vi "PostCopyScripting.vi"(10 "MetaDataObj":refnum<class "MetaDataObj.lvclass">, 11 "User Project":refnum<vi>) -> ()   [LabVIEW 2020, in "ADAS_IO_Template_MDO.lvclass"]
uses:
  ADAS_IO_Template_MDO.lvclass
  <resource>/dialog/NewProjectWizard/MetaDataObj/MetaDataObj.lvclass
  C:/Program Files/National Instruments/LabVIEW 2020/resource/dialog/NewProjectWizard/MetaDataObj/MetaDataObj.lvclass
  <resource>/dialog/NewProjectWizard/MetaDataObj/MetaDataObj.lvclass/MetaDataObj.ctl
  <resource>/dialog/NewProjectWizard/MetaDataObj/Accessors/Read Project Name.vi
  <resource>/dialog/NewProjectWizard/MetaDataObj/Accessors/Read Project Root.vi
  <resource>/dialog/NewProjectWizard/MetaDataObj/Accessors/Read Overlay Pixmap.vi
  <vilib>/LabVIEW Icon API/lv_icon/Classes/Icon/Icon.lvclass
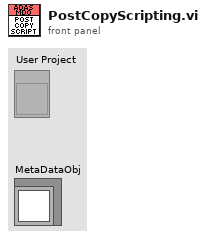
[diagram p1: front panel]
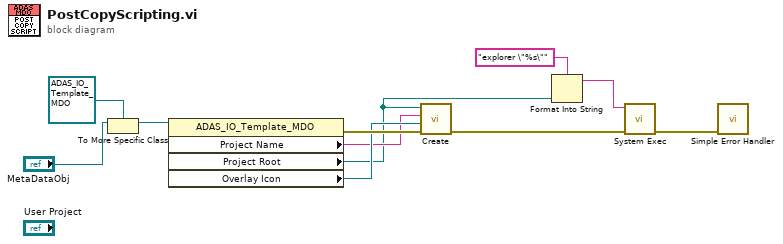
[diagram p0: block diagram]
diagram:
  n1 = To More Specific Class(target class=refnum<class "ADAS_IO_Template_MDO.lvclass"> refnum ("ADAS_IO_Template_MDO.lvclass"), reference="MetaDataObj") -> (specific class reference=w8:refnum<class "ADAS_IO_Template_MDO.lvclass">)  [unwired: 1 in, 1 out]
  n2 = property class="ADAS_IO_Template_MDO"(reference=w8) -> (error out=w11:errorcluster, "Project Name"=w6:string, "Project Root"=w3:path, "Overlay Icon"=w7:refnum<class "Icon.lvclass">)  [unwired: 1 in, 1 out]
  n3 = call "Create.vi"("error in (no error)"=w11, "Overlay Icon"=w7, "New Name"=w6, "Destination Directory"=w3) -> ("error out"=w1:errorcluster)  [unwired: 7 in]
  n4 = Format Into String(format string="explorer \"%s\"", w3) -> (resulting string=w4:string)  [unwired: 2 in, 1 out]
  n5 = call <vilib>:"System Exec.vi"("error in (no error)"=w1, "command line"=w4) -> ("error out"=w2:errorcluster)  [unwired: 6 in, 3 out]
  n6 = call <vilib>:"Simple Error Handler.vi"("error in (no error)"=w2) -> ()  [unwired: 4 in, 5 out]
